vi "UI Test.vi"() -> ()   [LabVIEW 2016]
panel:
  out "XY graph":cluster{"Wavenumber":dbl[], "Data":dbl[]}[](graph)
  out "Waveform Graph":dbl[](graph)
  out "XY Graph":cluster{"Intensity Data":dbl[], "Array":dbl[]}[](graph)
  out "Intensity Graph 2":dbl[][](graph)
  out "System XY Graph":cluster{dbl, dbl}[](graph)
  out "System Intensity Chart":dbl[][](graph)
  out "Intensity Graph":dbl[][](graph)
  # "JKI"
  # "System 2.0"
  # "Patrick Graph"
  # "Flatline:"
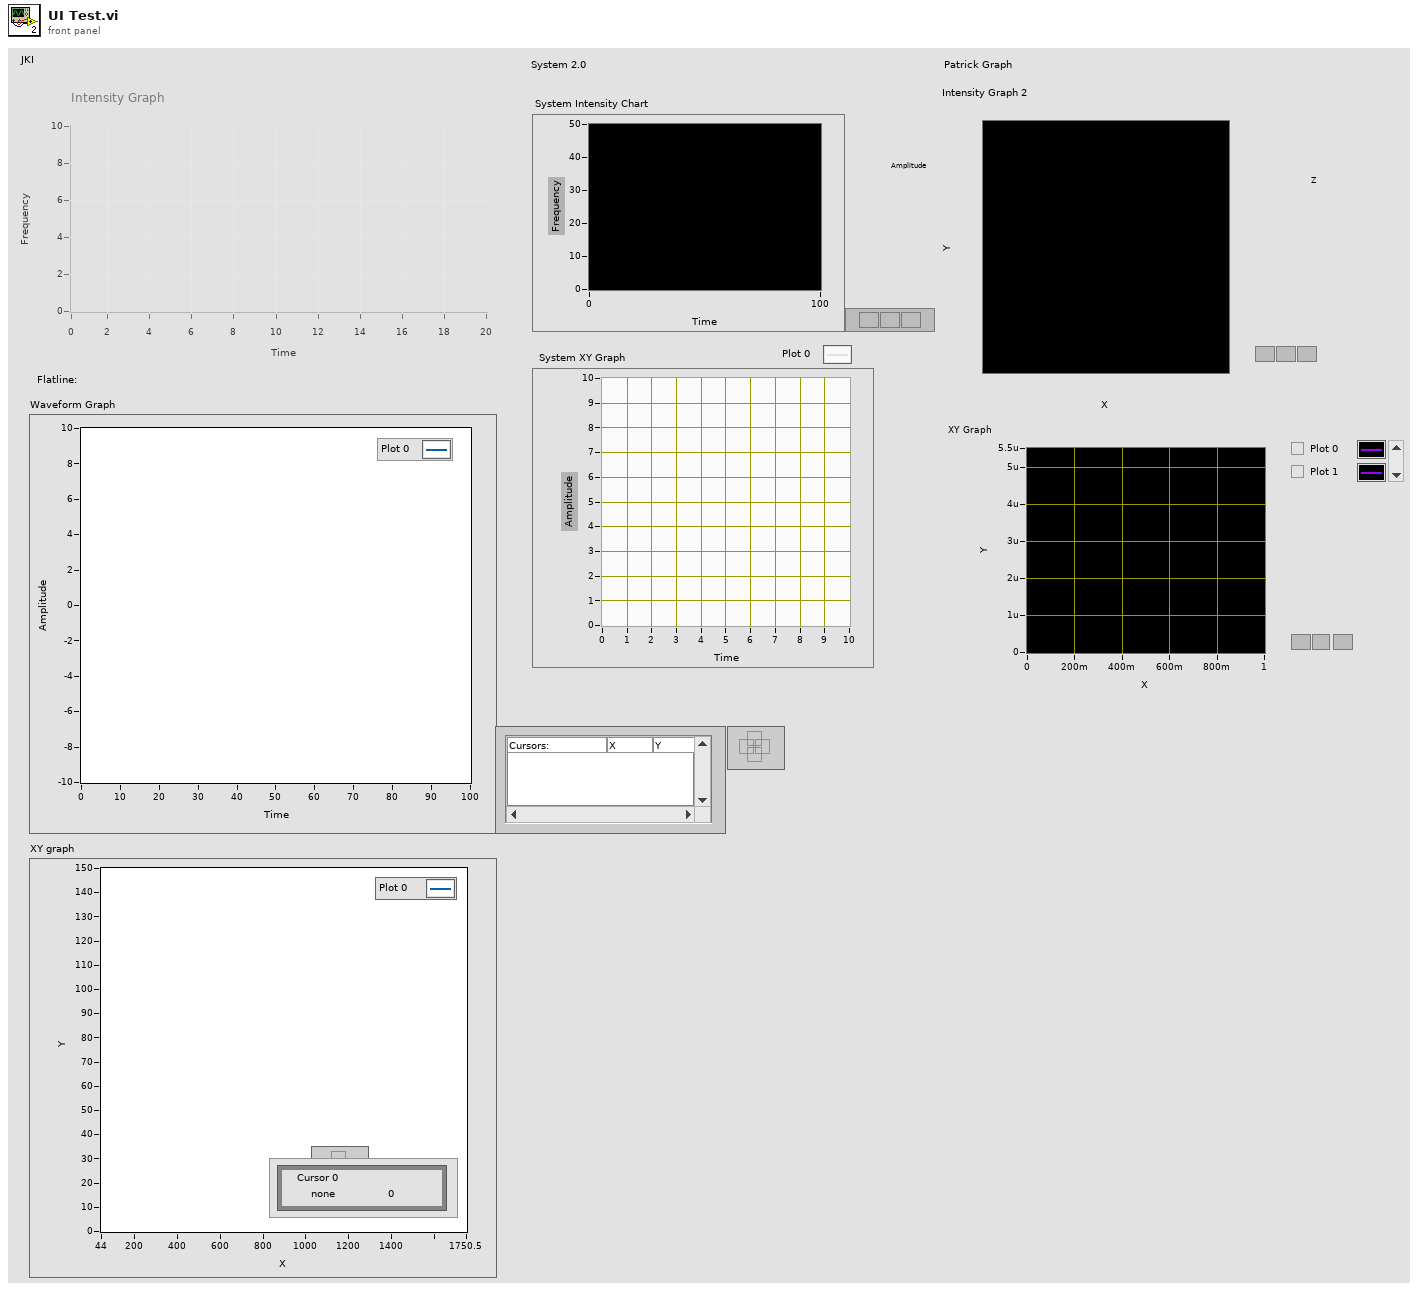
[diagram p1: front panel]
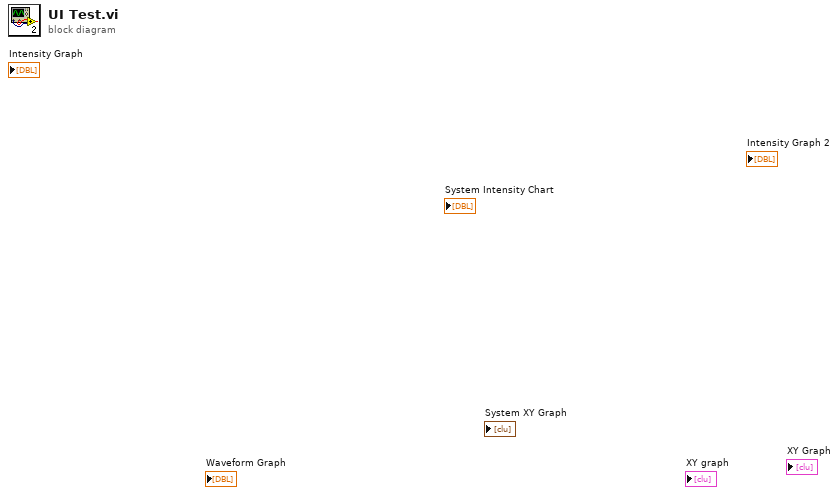
[diagram p0: block diagram]
diagram:
